vi "CurrentItem.vi"(0 "object in":refnum<class "BFSTreeIterator.lvclass">, 5 "Error In":errorcluster) -> (14 "object out":refnum<class "BFSTreeIterator.lvclass">, 16 "Current Item":refnum<class "Node.lvclass">, 19 "Error Out":errorcluster)   [LabVIEW 2024, in "BFSTreeIterator.lvclass"]
doc: "Returns current item according to traversal type"
uses:
  BFSTreeIterator.lvclass
  Node_class/Node.lvclass
  BFSTreeIterator.lvclass/BFSTreeIterator.ctl
panel:
  # "Connector Pane"
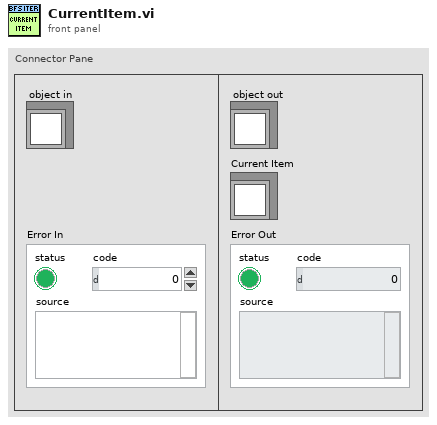
[diagram p1: front panel]
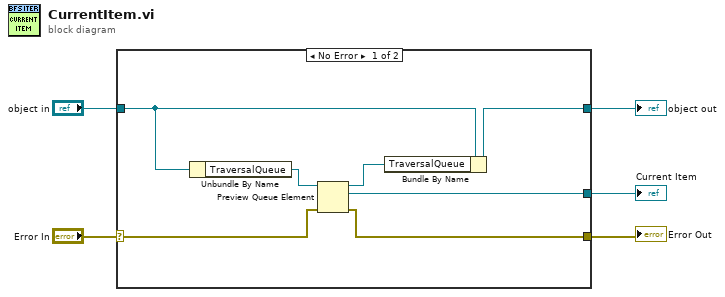
[diagram p0: block diagram]
diagram:
  n1 = case shown="No Error" "Error In" {
    selector: "Error In" -> [w7 w14]
    tunnel: [w6 w14] -> w4
    tunnel: [w9 w13] -> w2
    tunnel: "object in" -> [w12 w13]
    tunnel: [w10 _] -> w1
    frame No Error {
      n2 = Unbundle By Name(w12) -> ("TraversalQueue"=w11:refnum<queue>)
      n3 = Preview Queue Element(queue=w11, error in (no error)=w7) -> (queue out=w8:refnum<queue>, element=w10:refnum<class "Node.lvclass">, error out=w6:errorcluster)  [unwired: 1 in, 1 out]
      n4 = Bundle By Name(cluster=w12, "TraversalQueue"=w8) -> (w9:refnum<class "BFSTreeIterator.lvclass">)
    }
    frame Error {
    }
  }
  "Error Out" <- w4
  "object out" <- w2
  "Current Item" <- w1
